vi "Arrange GU Automatically.vi"(8 "error in":errorcluster, 11 "Curr Cal Cfg In":T1) -> (0 "error out":errorcluster, 3 "Curr Cal Cfg Out":T1)   [LabVIEW 2020, in "GUCalibration2.lvlib"]
uses:
  GUCalibration2.lvlib
  Controls/Config Data Type.ctl
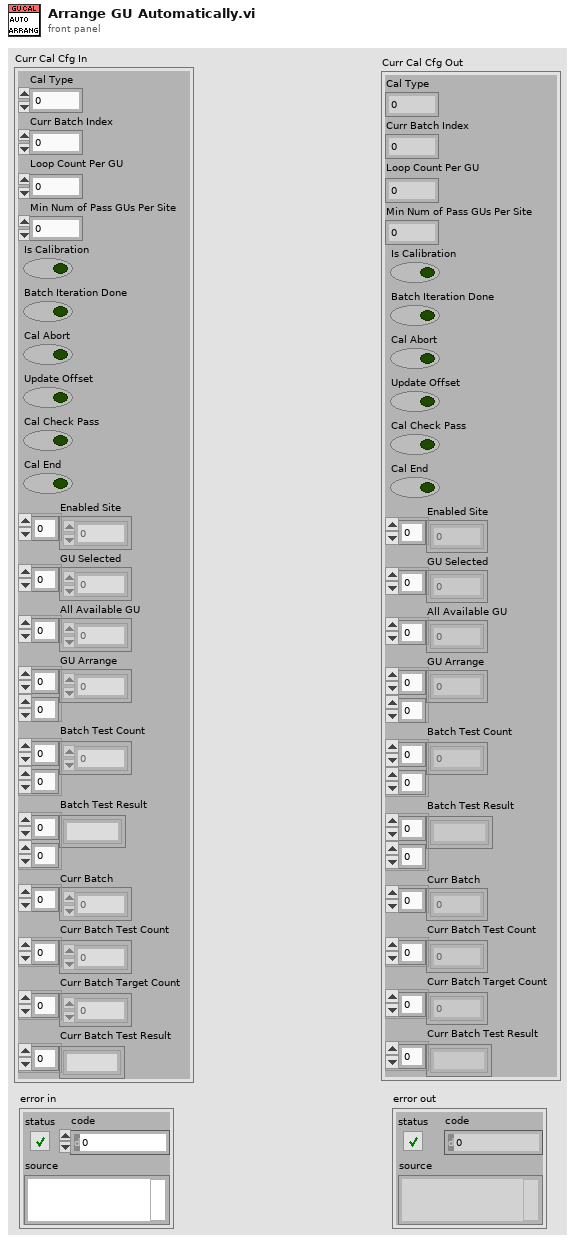
[diagram p1: front panel]
types:
  T1 = typedef "GUCalibration2.lvlib/Config Data Type.ctl" = cluster{"Cal Type":i32, "Curr Batch Index":i32, "Loop Count Per GU":i32, "Min Num of Pass GUs Per Site":i32, "Is Calibration":bool, "Batch Iteration Done":bool, "Cal Abort":bool, "Update Offset":bool, "Cal Check Pass":bool, "Cal End":bool, "Enabled Site":i32[], "GU Selected":i32[], "All Available GU":i32[], "GU Arrange":i32[][], "Batch Test Count":i32[][], "Batch Test Result":string[][], "Curr Batch":i32[], "Curr Batch Test Count":i32[], "Curr Batch Target Count":i32[], "Curr Batch Test Result":string[]}
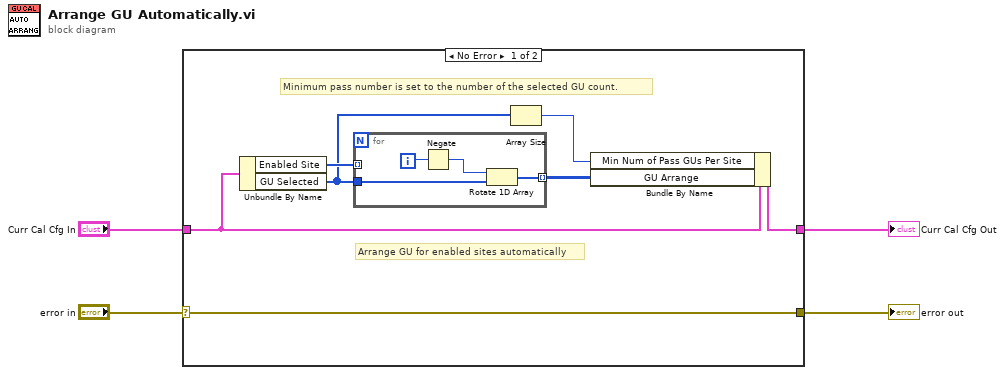
[diagram p0: block diagram]
diagram:
  n1 = case shown="No Error" "error in" {
    selector: "error in" -> [w9 w16]
    tunnel: [w9 w16] -> w4
    tunnel: [w10 _] -> w2
    tunnel: "Curr Cal Cfg In" -> [w11 _]
    frame No Error {
      # "Minimum pass number is set to the number of the selected GU count."
      # "Arrange GU for enabled sites automatically"
      n2 = Unbundle By Name(w11) -> ("Enabled Site"=w7:i32[], "GU Selected"=w5:i32[])
      n3 = for {
        tunnel: w5 -> [w15]
        tunnel: [w14] -> w8 mode=indexing
        tunnel: w7 -> [_] mode=indexing
        i -> [w13]
        n4 = Negate(x=w13) -> (-x=w12:i32)
        n5 = Rotate 1D Array(1:w15, 2:w12) -> (0:w14:i32[])
      }
      n6 = Array Size(array=w5) -> (size(s)=w6:i32)
      n7 = Bundle By Name(cluster=w11, "Min Num of Pass GUs Per Site"=w6, "GU Arrange"=w8) -> (w10:T1)
    }
    frame Error {
    }
  }
  "error out" <- w4
  "Curr Cal Cfg Out" <- w2
